vi "adapter_microphone.vi"(10 "configuration_microphone":T1={"chunk"=512, "profile"=3, "level"=41, "_reserved_0"=0, "_reserved_1"=0, "_reserved_2"=0, "_reserved_3"=0, "_reserved_4"=0, "_reserved_5"=0}, 11 "path in":path=path "hl2ss_ulm.dll") -> (2 "configuration":u64, 3 "path out":path)   [LabVIEW 2023]
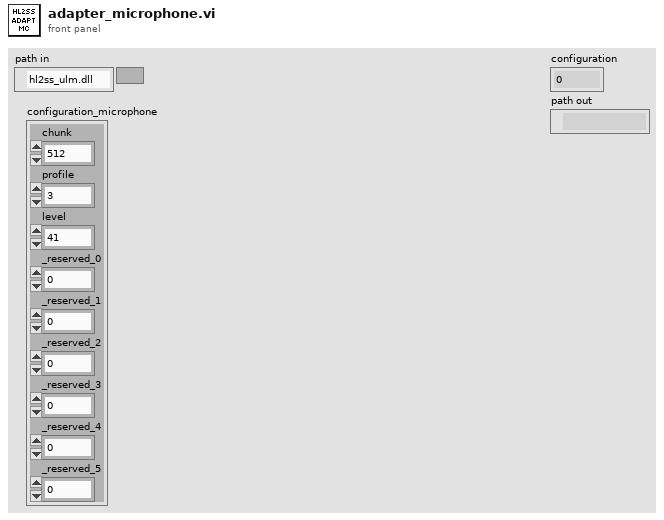
[diagram p1: front panel]
types:
  T1 = cluster{"chunk":u64, "profile":u8, "level":u8, "_reserved_0":u8, "_reserved_1":u8, "_reserved_2":u8, "_reserved_3":u8, "_reserved_4":u8, "_reserved_5":u8}
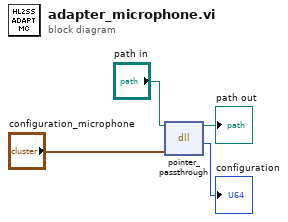
[diagram p0: block diagram]
diagram:
  n1 = dll-call lib="C:/Users/jcds/Documents/GitHub/hl2ss/extensions/client_labview/hl2ss_ulm.dll" fn="pointer_passthrough"(path in="path in", "p"="configuration_microphone") -> (path out=→"path out":path, "return type"=→"configuration":u64)  [unwired: 3 in, 1 out]
